vi "Logger.Add.vi"(8 "error in":errorcluster, 10 "All Slots":T1[](array[typedef]), 11 "Refnum in":refnum<k34>) -> (0 "error out":errorcluster, 1 "TS NOK":dbl[](array[numeric]), 2 "TS OK":dbl[](array[numeric]), 3 "Refnum out":refnum<k34>)   [LabVIEW 2016]
uses:
  Sequence/Sequence.Test.Status.ctl
  Sequence/Sequence.Slot.StatusData.ctl
  Sequence/Sequence.Test.Unload.Status.ctl
  Sequence/Sequence.Prod.StatusData.ctl
  Sequence/Sequence.Step.Status.ctl
  Sequence/Sequence.Test.BreakReason.ctl
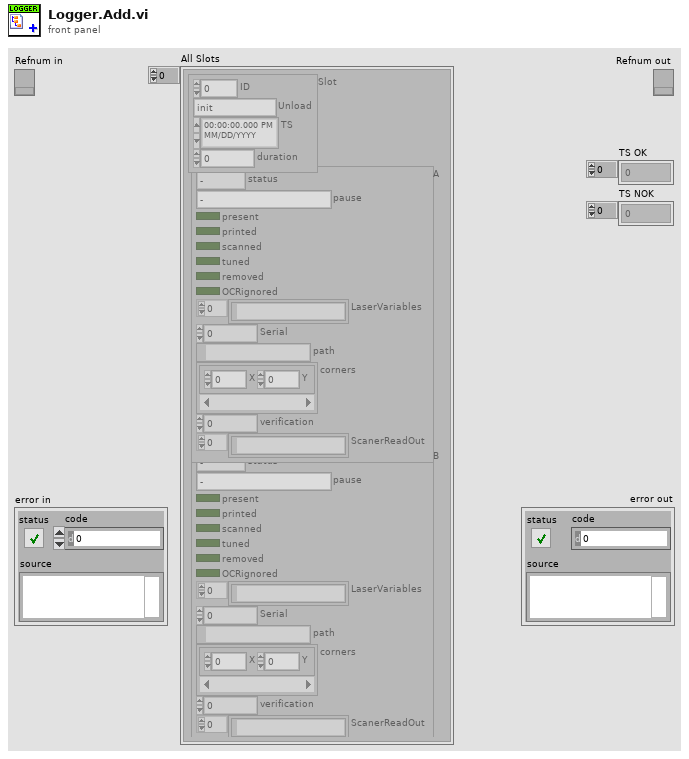
[diagram p1: front panel]
types:
  T1 = typedef "Sequence.Test.Status.ctl" = cluster{"Slot":T2, "A":T4, "B":T4}
  T2 = typedef "Sequence.Slot.StatusData.ctl" = cluster{"ID":i32, "Unload":T3, "TS":timestamp, "duration":u32}
  T3 = typedef "Sequence.Test.Unload.Status.ctl" = enum16{"init", "check NOK", "check OK", "wait on NOK", "wait on OK", "wait on Unload", "done"}
  T4 = typedef "Sequence.Prod.StatusData.ctl" = cluster{"status":T5, "pause":T6, "present":bool, "printed":bool, "scanned":bool, "tuned":bool, "removed":bool, "OCRignored":bool, "LaserVariables":string[], "Serial":i32, "path":path, "corners":cluster{"X":i32, "Y":i32}[], "verification":u8, "ScanerReadOut":string[]}
  T5 = typedef "Sequence.Step.Status.ctl" = enum16{"-", "Pending", "Running", "Skipped", "Passed", "Failed", "Done", "Error", "Aborted", "Stopped"}
  T6 = typedef "Sequence.Test.BreakReason.ctl" = enum16{"-", "NOK container", "OK container", "Rev empty", "Rev missing", "Rev wrong", "Fork missing", "Fork wrong", "NOK limit", "Unload failure", "Single slot", "Part done", "Err: Prod move work", "Err: Prod move home", "Err: Prod lift work", "Err: Prod lift home", "Err: Prod Arm Work", "Err: Prod Arm NOK", "Err: Prod Arm OK", "Err: Prod NOK suck", "Err: Prod NOK drop", "Err: Prod OK missing", "Err: Prod OK suck", "Err: Prod OK drop"}
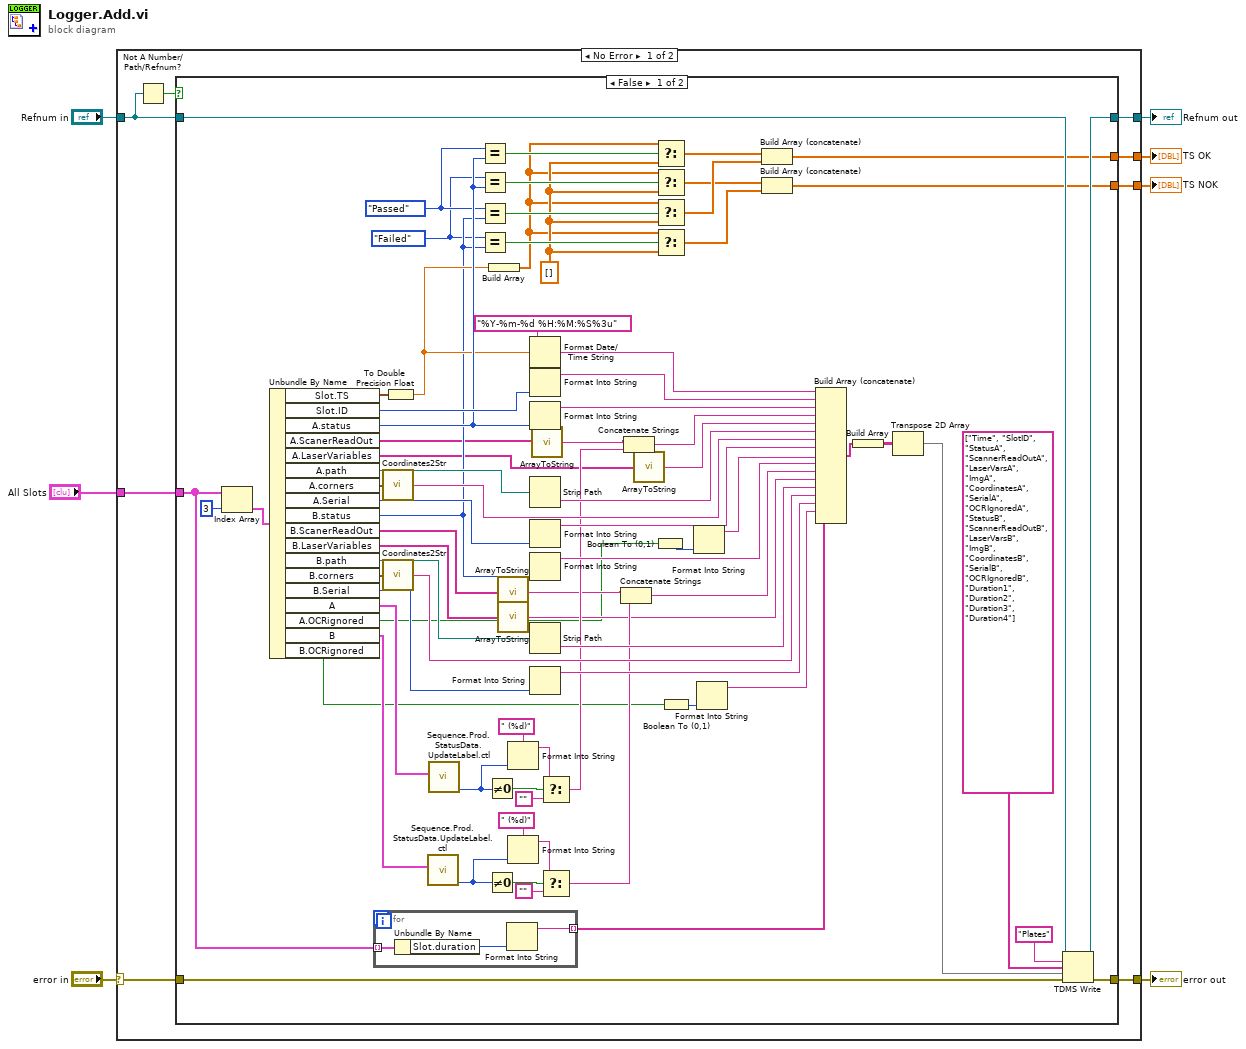
[diagram p0: block diagram]
diagram:
  n1 = case shown="No Error" "error in" {
    selector: "error in" -> [w15 w101]
    tunnel: [w13 w100] -> w7
    tunnel: [w14 w101] -> w6
    tunnel: "Refnum in" -> [w12 w100]
    tunnel: "All Slots" -> [w10 _]
    tunnel: [w9 _] -> w3
    tunnel: [w8 _] -> w2
    frame No Error {
      n2 = Not A Number/Path/Refnum?(number/path/refnum=w12) -> (NaN/Path/Refnum?=w11:bool)
      n3 = case shown="False" w11 {
        tunnel: w15 -> [w90 w98]
        tunnel: [w92 w98] -> w14
        tunnel: [w93 w99] -> w13
        tunnel: w12 -> [w94 w99]
        tunnel: w10 -> [w31 _]
        tunnel: [w54 _] -> w9
        tunnel: [w53 _] -> w8
        frame False {
          w51 = Sequence.Step.Status."Failed" ("x")
          w52 = Sequence.Step.Status."Passed" ("x")
          w62 = dbl[] [] ("f")
          n4 = Index Array(array=w31, index=3) -> (element=w33:T1)
          n5 = Unbundle By Name(w33) -> ("Slot.TS"=w68:timestamp, "Slot.ID"=w77:i32, "A.status"=w69:T5, "A.ScanerReadOut"=w26:string[], "A.LaserVariables"=w30:string[], "A.path"=w83:path, "A.corners"=w80:cluster{"X":i32, "Y":i32}[], "A.Serial"=w76:i32, "B.status"=w65:T5, "B.ScanerReadOut"=w24:string[], "B.LaserVariables"=w28:string[], "B.path"=w74:path, "B.corners"=w73:cluster{"X":i32, "Y":i32}[], "B.Serial"=w72:i32, "A"=w49:T4, "A.OCRignored"=w22:bool, "B"=w48:T4, "B.OCRignored"=w18:bool)
          n6 = for {
            tunnel: w31 -> [w97] mode=indexing
            tunnel: [w95] -> w16 mode=indexing
            n7 = Unbundle By Name(w97) -> ("Slot.duration"=w96:u32)
            n8 = Format Into String(w96) -> (resulting string=w95:string)  [unwired: 3 in, 1 out]
          }
          n9 = call "Coordinates2Str.vi"("Coordinates"=w80) -> ("String"=w79:string)  [unwired: 1 in]
          n10 = call "Coordinates2Str.vi"("Coordinates"=w73) -> ("String"=w78:string)  [unwired: 1 in]
          n11 = To Double Precision Float(number=w68) -> (double precision float=w67:dbl)
          n12 = call "Sequence.Prod.StatusData.UpdateLabel.ctl"("Slot"=w48) -> ("Status"=w36:i32)  [unwired: 9 in, 1 out]
          n13 = call "Sequence.Prod.StatusData.UpdateLabel.ctl"("Slot"=w49) -> ("Status"=w46:i32)  [unwired: 9 in, 1 out]
          n14 = Equal?(x=w52, y=w69) -> (x = y?=w70:bool)
          n15 = Equal?(x=w51, y=w69) -> (x = y?=w66:bool)
          n16 = Equal?(x=w52, y=w65) -> (x = y?=w64:bool)
          n17 = Equal?(x=w51, y=w65) -> (x = y?=w63:bool)
          n18 = Not Equal To 0?(x=w46) -> (x != 0?=w47:bool)
          n19 = Not Equal To 0?(x=w36) -> (x != 0?=w37:bool)
          n20 = Build Array(w67) -> (w61:dbl[])
          n21 = call "ArrayToString.vi"("Array"=w24) -> ("string"=w23:string)
          n22 = call "ArrayToString.vi"("Array"=w28) -> ("string"=w27:string)
          n23 = Format Into String(format string=" (%d)", w46) -> (resulting string=w44:string)  [unwired: 2 in, 1 out]
          n24 = Format Into String(format string=" (%d)", w36) -> (resulting string=w39:string)  [unwired: 2 in, 1 out]
          n25 = Format Date/Time String(time format string (%c)="%Y-%m-%d %H:%M:%S%3u", seconds (now)=w67) -> (date/time string=w59:string)  [unwired: 1 in]
          n26 = Format Into String(w77) -> (resulting string=w60:string)  [unwired: 3 in, 1 out]
          n27 = Format Into String(w69) -> (resulting string=w86:string)  [unwired: 3 in, 1 out]
          n28 = Strip Path(path=w83) -> (name=w82:string)  [unwired: 1 out]
          n29 = Format Into String(w76) -> (resulting string=w75:string)  [unwired: 3 in, 1 out]
          n30 = Format Into String(w65) -> (resulting string=w85:string)  [unwired: 3 in, 1 out]
          n31 = Strip Path(path=w74) -> (name=w81:string)  [unwired: 1 out]
          n32 = Format Into String(w72) -> (resulting string=w71:string)  [unwired: 3 in, 1 out]
          n33 = call "ArrayToString.vi"("Array"=w26) -> ("string"=w25:string)
          n34 = Select(t=w44, s=w47, f="") -> (s? t:f=w41:string)
          n35 = Select(t=w39, s=w37, f="") -> (s? t:f=w35:string)
          n36 = Concatenate Strings(w23, w35) -> (w40:string)
          n37 = Concatenate Strings(w25, w41) -> (w42:string)
          n38 = call "ArrayToString.vi"("Array"=w30) -> ("string"=w29:string)
          n39 = Boolean To (0,1)(Boolean=w22) -> (0, 1=w21:i16)
          n40 = Select(t=w61, s=w70, f=w62) -> (s? t:f=w58:dbl[])
          n41 = Select(t=w61, s=w66, f=w62) -> (s? t:f=w56:dbl[])
          n42 = Select(t=w61, s=w64, f=w62) -> (s? t:f=w57:dbl[])
          n43 = Select(t=w61, s=w63, f=w62) -> (s? t:f=w55:dbl[])
          n44 = Boolean To (0,1)(Boolean=w18) -> (0, 1=w19:i16)
          n45 = Format Into String(w21) -> (resulting string=w20:string)  [unwired: 3 in, 1 out]
          n46 = Format Into String(w19) -> (resulting string=w17:string)  [unwired: 3 in, 1 out]
          n47 = Build Array (concatenate)(w58, w57) -> (w54:dbl[])
          n48 = Build Array (concatenate)(w56, w55) -> (w53:dbl[])
          n49 = Build Array (concatenate)(w59, w60, w86, w42, w29, w82, w79, w75, w20, w85, w40, w27, w81, w78, w71, w17, w16) -> (w91:string[])
          n50 = Build Array(w91) -> (w87:string[][])
          n51 = Transpose 2D Array(2D array=w87) -> (transposed array=w84:string[][])
          n52 = TDMS Write(0:w94, 5:"Plates" ("group name in (Untitled)"), 7:string[] ["Time", "SlotID", "StatusA", "ScannerReadOutA", "LaserVarsA", "ImgA", "CoordinatesA", "SerialA", "OCRIgnoredA", "StatusB", "ScannerReadOutB", "LaserVarsB", "ImgB", "CoordinatesB", "SerialB", "OCRIgnoredB", "Duration1", "Duration2", "Duration3", "Duration4"] ("channel name(s) in (Untitled)"), 9:w84, 11:w90) -> (4:w93:refnum<k34>, 15:w92:errorcluster)  [unwired: 1 in, 2 out]
        }
        frame True {
        }
      }
    }
    frame Error {
    }
  }
  "Refnum out" <- w7
  "error out" <- w6
  "TS OK" <- w3
  "TS NOK" <- w2
